vi "Send Command.vi"(7 "VolatusAPI":refnum<class "VolatusAPI.lvclass">, 8 "error in (no error)":errorcluster, 10 "Value":bool, 11 "2WayValve in":refnum<class "2WayValveV.lvclass">) -> (0 "error out":errorcluster, 3 "2WayValve out":refnum<class "2WayValveV.lvclass">)   [LabVIEW 2020, in "VolatusGUIElements.lvlib" / "2WayValveV.lvclass"]
uses:
  2WayValveV.lvclass
  Volatus/VolatusAPI/VolatusAPI.lvclass
  2WayValveV.lvclass/2WayValveV.ctl
  messages/CmdDigital/Class/Msg.lvclass/Msg.ctl
  Volatus/VolatusAPI/VolatusAPI.lvclass/VolatusAPI.ctl
  messages/CmdDigital/Class/Msg.lvclass
  C:/dev/lv20CE/relink/lv-protoc/LV-Proto/Message/Message.lvclass
  lv-vecto/Vecto/TCPMessageService/Send Message.vi
  <vilib>/Utility/error.llb/Error Cluster From Error Code.vi
  lv-protoc/LV-Proto/Message/Message.lvclass
  C:/dev/lv20CE/relink/lv-volatus/messages/CmdDigital/Class/Msg.lvclass
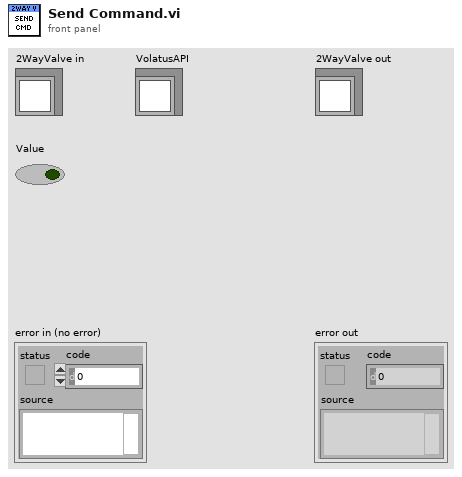
[diagram p1: front panel]
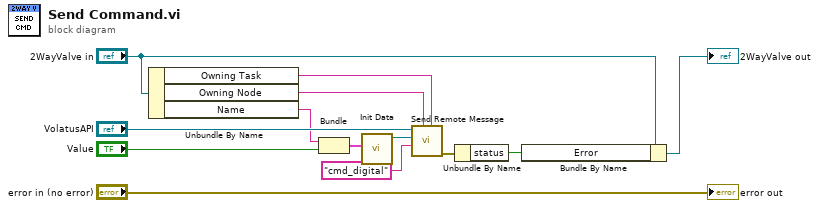
[diagram p0: block diagram]
diagram:
  n1 = Unbundle By Name("2WayValve in") -> ("Owning Task"=w10:string, "Owning Node"=w11:string, "Name"=w9:string)
  n2 = Bundle("Name"=w9, "Value"="Value") -> (w7:cluster{"Name":string, "Value":bool})  [unwired: 1 in]
  n3 = call "Init Data.vi"("Data"=w7) -> ("Msg out"=w6:refnum<class "Msg.lvclass">)  [unwired: 10 in]
  n4 = call "Send Remote Message.vi"("Target Task (None)"=w10, "Target Node"=w11, "Message Type"="cmd_digital", "Message"=w6, "VolatusAPI in"="VolatusAPI") -> ("error out"=w3:errorcluster)  [unwired: 5 in, 1 out]
  n5 = Unbundle By Name(w3) -> ("status"=w2:bool)
  n6 = Bundle By Name(cluster="2WayValve in", "Error"=w2) -> (→"2WayValve out":refnum<class "2WayValveV.lvclass">)
  "error out" <- "error in (no error)"
